vi "Description_parameter_type_telem_(SubVI).vi"(8 "error in (no error)":errorcluster, 11 "paramUnicorn in":T1) -> (0 "error out":errorcluster, 3 "paramUnicornIn out 2":T1)   [LabVIEW 2017, in "LV_Unicorn.lvlib"]
uses:
  LV_Unicorn.lvlib
  Control/unicorn_Param.ctl
  Control/unicorn_conn.ctl
  Control/unicorn_JSON.ctl
  Control/unicorn_ParamInt.ctl
  Control/unicorn_Telemetry.ctl
  Control/unicorn_Table.ctl
  Control/unicorn_ParamFloat.ctl
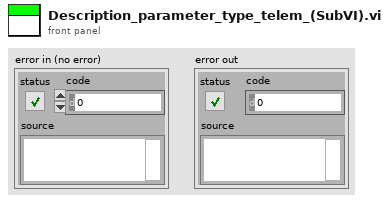
[diagram p1: front panel]
types:
  T1 = typedef "LV_Unicorn.lvlib/unicorn_Param.ctl" = cluster{"conParam":T2, "Param":T3}
  T2 = typedef "LV_Unicorn.lvlib/unicorn_conn.ctl" = cluster{"ReadIntParam":bool, "ReadDescrParam":bool, "ReadFloatParam":bool, "debug":bool, "ReadJSON":bool, "IP_address":string, "N_attempts":i32, "type_con":enum16{"Serial", "TCP"}, "MB_address":i32, "VISA":refnum<visa-resource-name>, "connection ID":refnum<k5>, "nameDevices":string, "timeout":i32, "port":u16, "type_version":string, "baud_rate":u32, "VersionControl":bool, "TCP_conn":bool, "WindowSize":i32}
  T3 = typedef "LV_Unicorn.lvlib/unicorn_JSON.ctl" = cluster{"NumParam":cluster{"NTelem":i32, "NInt":i32, "NFloat":i32, "NTable":i32}, "ParamInt":T4, "Telemetry":T5, "Table":T6, "ParamFloat":T7}
  T4 = typedef "LV_Unicorn.lvlib/unicorn_ParamInt.ctl" = cluster{"ID":string, "Num":i32, "Name":string, "Type":string, "Enum":string, "Desc":string, "Unit":string, "Access":string, "FormatStr":string, "Min":i32, "Max":i32}[]
  T5 = typedef "LV_Unicorn.lvlib/unicorn_Telemetry.ctl" = cluster{"ID":string, "Num":i32, "Name":string, "Desc":string, "Unit":string, "FormatStr":string, "Min":i32, "Max":i32}[]
  T6 = typedef "LV_Unicorn.lvlib/unicorn_Table.ctl" = cluster{"Num":i32, "Access":string, "ColumnCount":i32, "NeedParamPrepare":bool, "Columns":cluster{"Column":i32, "Desc":string, "Name":string}[], "DataType":string, "FormatStr":string, "ID":string, "Name":string, "RowCount":i32, "Rows":cluster{"Desc":string, "ID":string, "Max":i32, "Min":i32, "Name":string, "Row":i32, "Unit":string}[], "Type":string}[]
  T7 = typedef "LV_Unicorn.lvlib/unicorn_ParamFloat.ctl" = cluster{"ID":string, "Num":i32, "Name":string, "Type":string, "Enum":string, "Desc":string, "Unit":string, "Access":string, "FormatStr":string, "Min":sgl, "Max":sgl}[]
  T8 = typedef "unicorn_DescriptParam.ctl" = cluster{"Имя параметра":string, "Единица измерения":string, "Форматная строка ":string, "Уникальное имя":string, "Диапазон измерений":string, "lo":variant, "hi":variant, "Access":string}
  T9 = cluster{"ID":string, "Num":i32, "Name":string, "Desc":string, "Unit":string, "FormatStr":string, "Min":i32, "Max":i32}
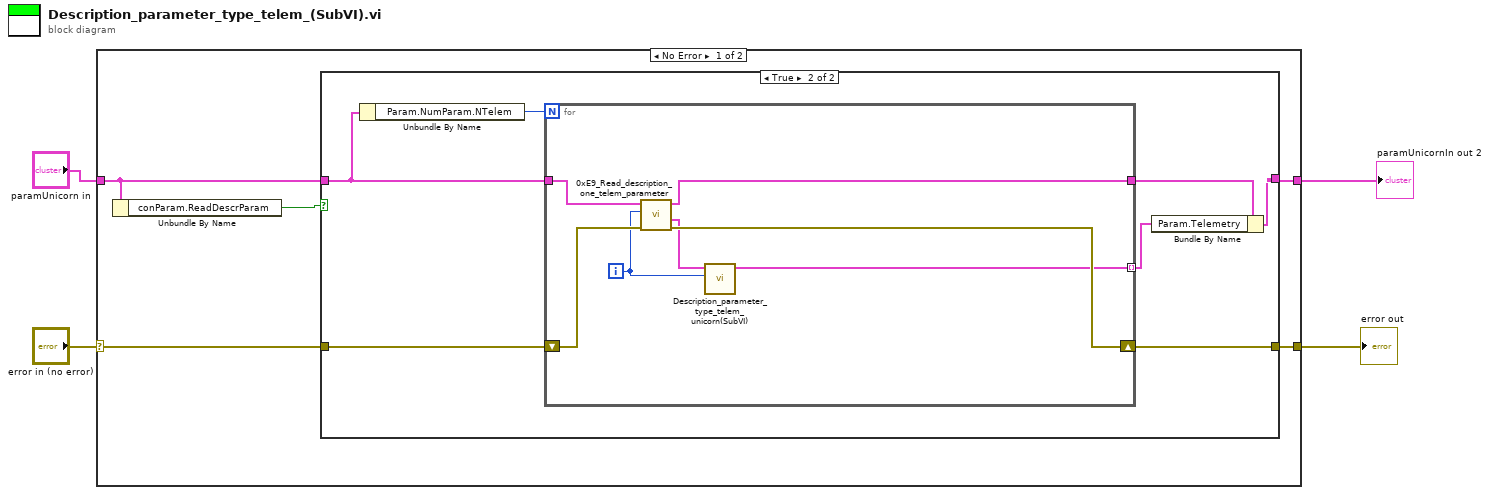
[diagram p0: block diagram]
diagram:
  n1 = case shown="No Error" "error in (no error)" {
    selector: "error in (no error)" -> [w8 w26]
    tunnel: [w9 w26] -> w4
    tunnel: [w7 w27] -> w3
    tunnel: "paramUnicorn in" -> [w6 w27]
    frame No Error {
      n2 = Unbundle By Name(w6) -> ("conParam.ReadDescrParam"=w5:bool)
      n3 = case shown="True" w5 {
        tunnel: [w10 w18] -> w9
        tunnel: w8 -> [w10 w17]
        tunnel: w6 -> [w11 w16]
        tunnel: [w11 w12] -> w7
        frame False {
        }
        frame True {
          n4 = Unbundle By Name(w16) -> ("Param.NumParam.NTelem"=w15:i32)
          n5 = for {
            N: w15 -> [_]
            shift-right: [w25] -> w18
            shift-left: w17 -> [w23]
            tunnel: [w19] -> w13 mode=indexing
            tunnel: w16 -> [w24]
            tunnel: [w22] -> w14
            i -> [w21]
            n6 = call "0xE9_Read_description_one_telem_parameter.vi"("error in (no error)"=w23, "NumberTelemParam"=w21, "paramUnicornIn in"=w24) -> ("error out"=w25:errorcluster, "Param"=w20:T8, "paramUnicornIn out 2"=w22:T1)  [unwired: 6 in]
            n7 = call "Description_parameter_type_telem_unicorn(SubVI).vi"("Numeric"=w21, "Param"=w20) -> ("output cluster"=w19:T9)  [unwired: 9 in]
          }
          n8 = Bundle By Name(cluster=w14, "Param.Telemetry"=w13) -> (w12:T1)
        }
      }
    }
    frame Error {
    }
  }
  "error out" <- w4
  "paramUnicornIn out 2" <- w3
